vi "Acquisition Message Loop.vi"(8 "error in (no error)":errorcluster, 9 "queue out":refnum<queue>, 10 "Data Notifier":refnum<notifier>, 11 "Message Queues":T1) -> (0 "error out":errorcluster)   [LabVIEW 2018, in "Acquisition.lvlib"]
doc: "Message loop for handling messages pertaining to the acquisition of data from the hardware."
uses:
  Acquisition.lvlib
  support/Message Queue/Message Cluster.ctl
  Acquisition State.ctl
  GlobalVariable/GlobalDisconnected.vi
  GlobalVariable/GlobalFirstRep.vi
  GlobalVariable/GlobalPowerByTime.vi
  GlobalVariable/GlobalPosXbyTime.vi
  GlobalVariable/GlobalPosYbyTime.vi
  GlobalVariable/GlobalProfileByTime.vi
  GlobalVariable/GlobalTensionByTime.vi
  GlobalVariable/GlobalTemperatureByTime.vi
  GlobalVariable/GlobalPredictedPower.vi
  GlobalVariable/Globalt0.vi
  support/Message Queue/Enqueue Message (Single).vi
  GlobalVariable/GlobalLongueurOnde.vi
  GlobalVariable/GlobalTimeStep.vi
  <vilib>/Utility/error.llb/Error Cluster From Error Code.vi
  <vilib>/ErrorRing/Error Ring.xnode
  support/Message Queue/Message Queue.lvlib
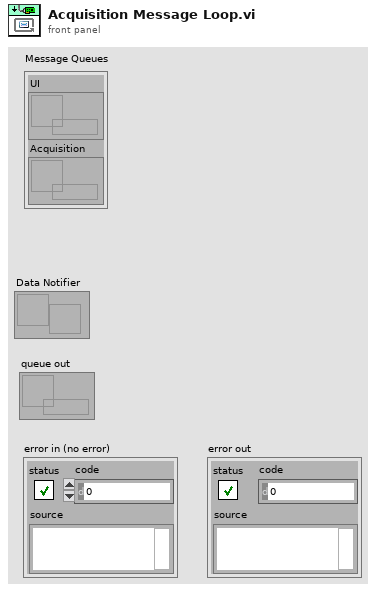
[diagram p1: front panel]
types:
  T1 = cluster{"UI":refnum<queue>, "Acquisition":refnum<queue>}
  T2 = typedef "Acquisition.lvlib/Acquisition State.ctl" = enum16{"Idle", "Acquiring"}
  T3 = enum16{"open", "replace", "create", "open or create", "replace or create", "replace or create with confirmation"}
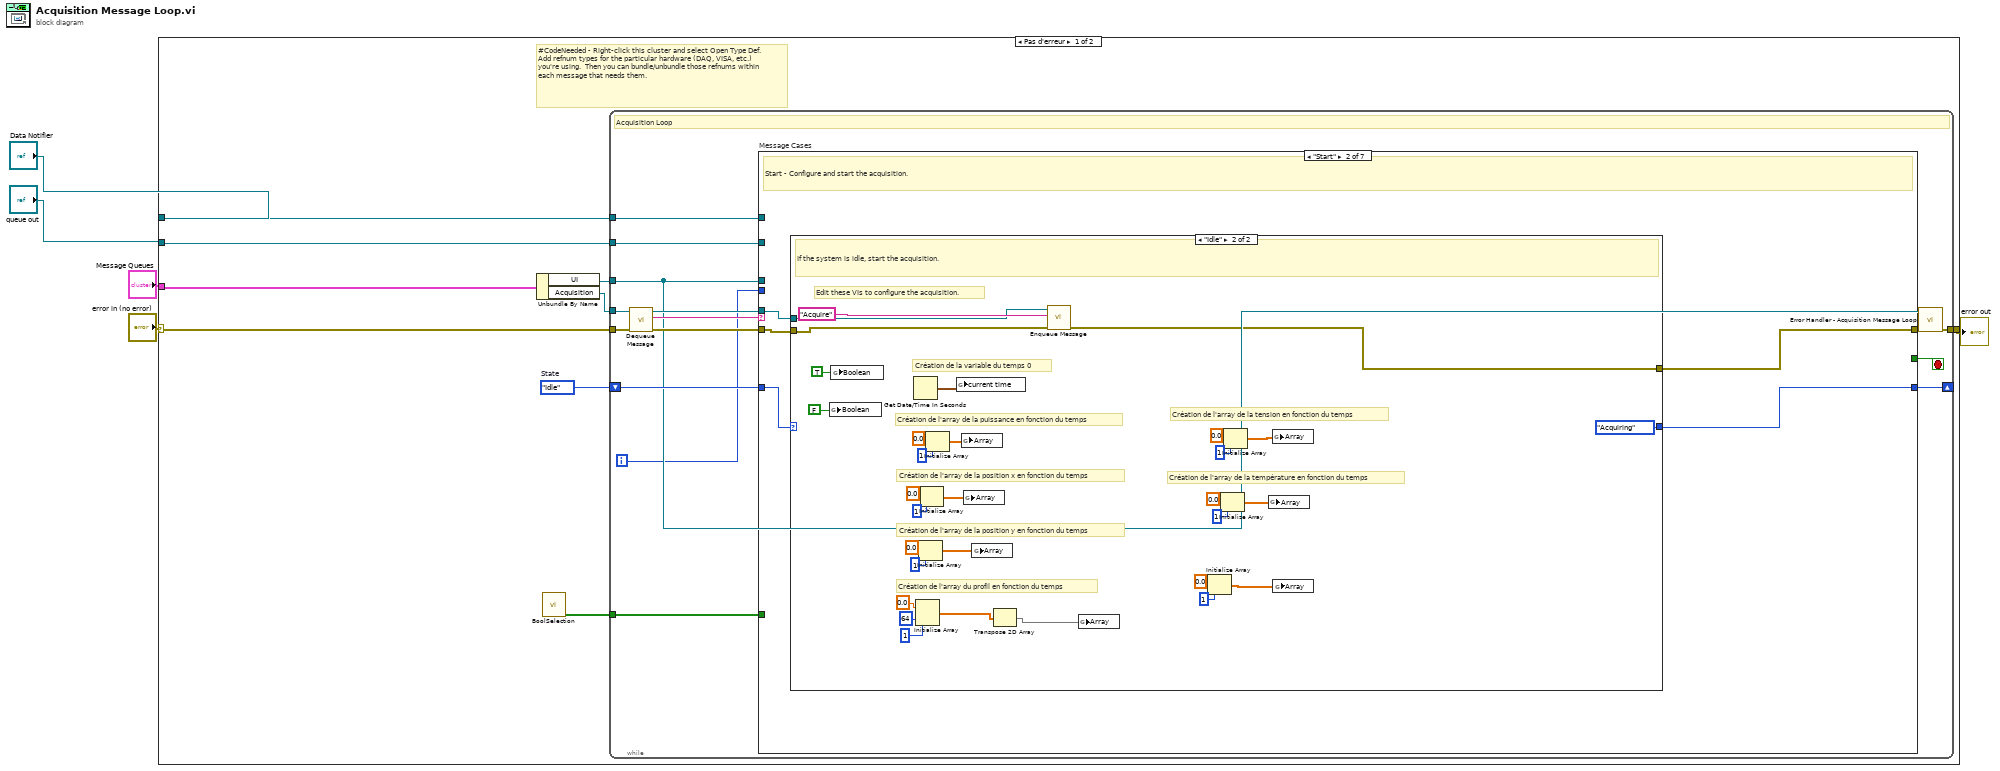
[diagram p0: block diagram]
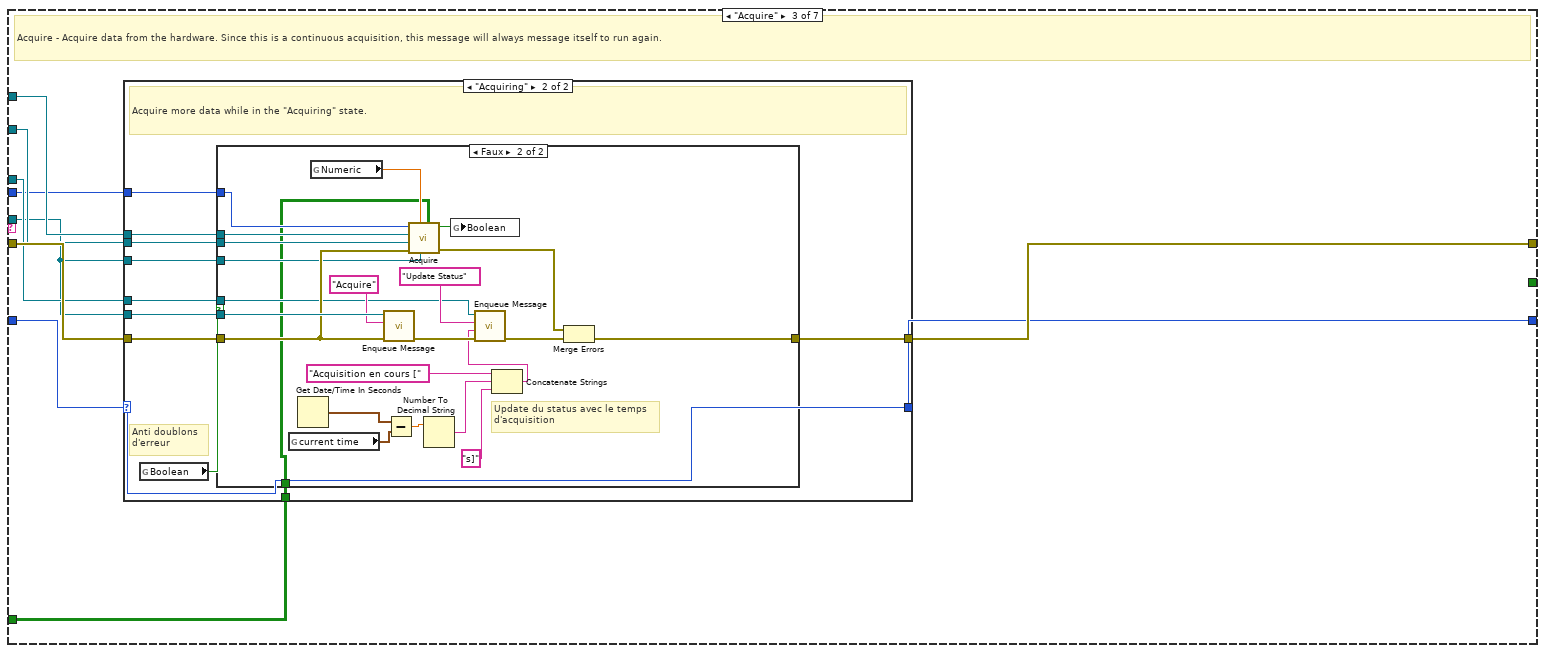
[diagram p4: hidden frame]
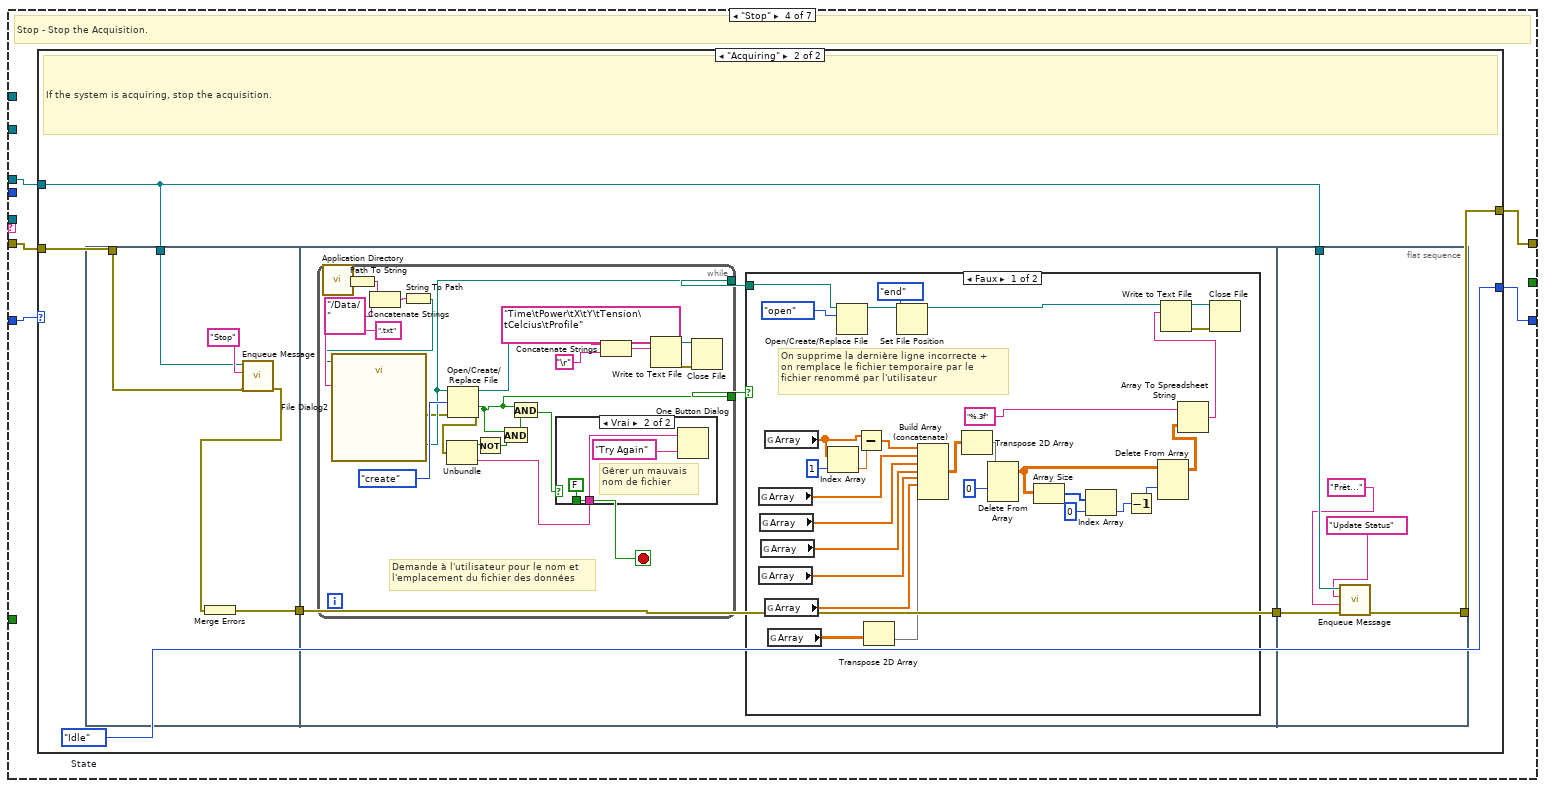
[diagram p7: hidden frame]
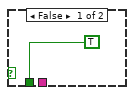
[diagram p10: hidden frame]
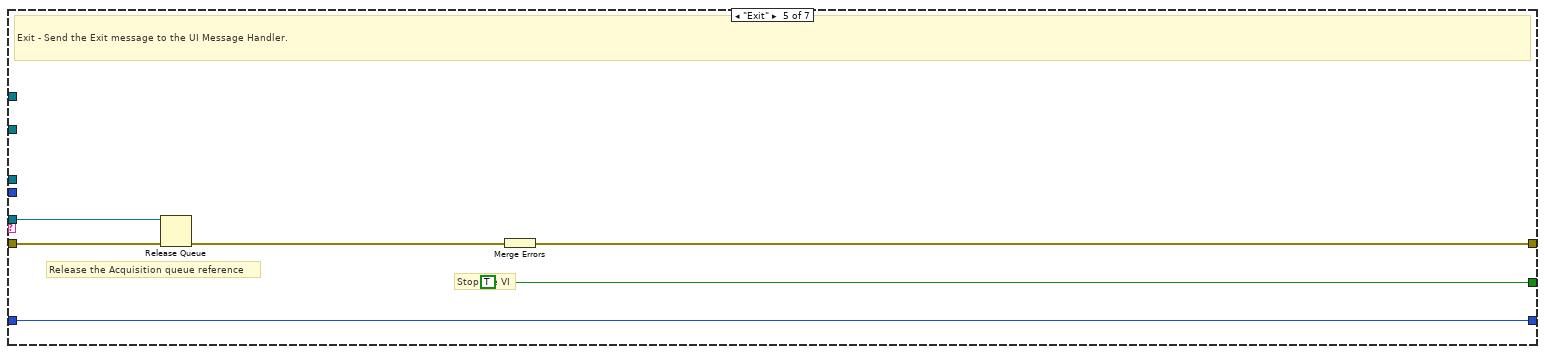
[diagram p11: hidden frame]
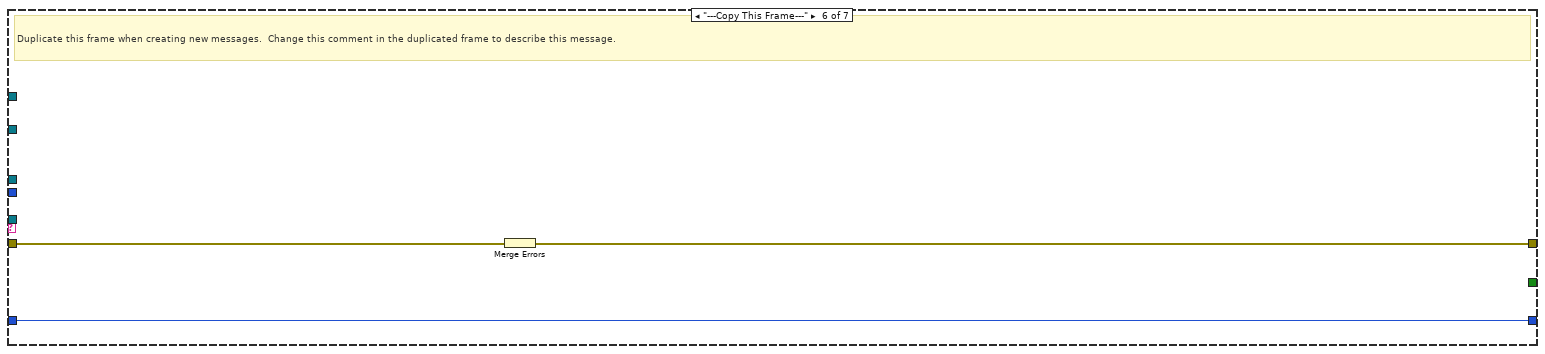
[diagram p12: hidden frame]
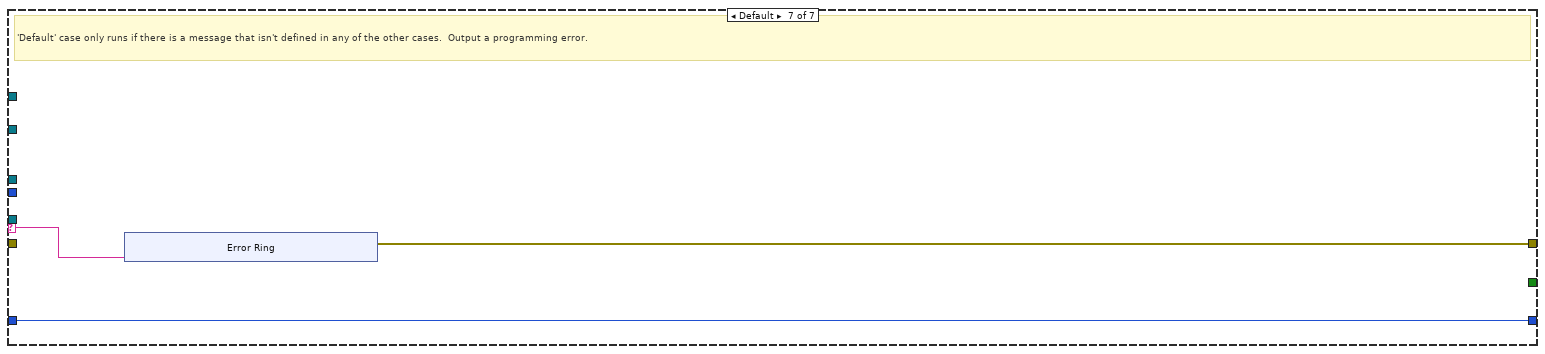
[diagram p13: hidden frame]
diagram:
  n1 = case shown="Pas d'erreur" "error in (no error)" {
    selector: "error in (no error)" -> [w11 w218]
    tunnel: "Message Queues" -> [w14 _]
    tunnel: [w12 w218] -> w4
    tunnel: "Data Notifier" -> [w9 _]
    tunnel: "queue out" -> [w8 _]
    frame No Error {
      w7 = Acquisition_State."Idle"  # State
      # "#CodeNeeded - Right-click this cluster and select Open Type Def.  Add refnum types for the particular hardware (DAQ, VISA, etc.) you're using.  Then you can bundle/unbundle those refnums within each message that needs them."
      n2 = Unbundle By Name(w14) -> ("UI"=w10:refnum<queue>, "Acquisition"=w13:refnum<queue>)
      n3 = call "BoolSelection.vi"() -> ("BoolSelection"=w6:bool[][])  [unwired: 11 in]
      n4 = while {
        tunnel: w13 -> [w17]
        tunnel: w10 -> [w18]
        tunnel: w9 -> [w25]
        tunnel: w8 -> [w24]
        shift-right: [w22] -> _
        shift-left: w7 -> [w23]
        tunnel: w11 -> [w28]
        tunnel: [w21] -> w12
        tunnel: w6 -> [w15]
        i -> [w16]
        stop <- w29 stop-if-true
        # "Acquisition Loop"
        n5 = call "Dequeue Message.vi"("error in (no error)"=w28, "Message Queue"=w17) -> ("error out"=w27:errorcluster, "Message"=w26:string, "dup Message Queue"=w19:refnum<queue>)  [unwired: 6 in, 1 out]
        n6 = case "Message Cases" shown="\"Start\"" w26 {
          selector: w26 -> [_ _ _ _ _ _ w208]
          tunnel: w19 -> [_ w34 w72 _ w200 _ _]
          tunnel: w27 -> [w31 w35 w78 w120 w202 w207 _]
          tunnel: [w31 w36 w79 w118 w203 w206 w209] -> w20
          tunnel: [_ _ _ _ TRUE _ _] -> w29
          tunnel: w18 -> [_ _ w73 w119 _ _ _]
          tunnel: w25 -> [_ _ w77 _ _ _ _]
          tunnel: w24 -> [_ _ w76 _ _ _ _]
          tunnel: w23 -> [w30 w32 w74 w121 w199 w205 w210]
          tunnel: [w30 w33 w75 w117 w199 w205 w210] -> w22
          tunnel: w16 -> [_ _ w71 _ _ _ _]
          tunnel: w15 -> [_ _ w70 _ _ _ _]
          frame "Initialize" {
            # "Initialize  - Initialize is currently a no-op.  The hardware initialization takes place in the 'Start' message."
          }
          frame "Start" {
            # "Start - Configure and start the acquisition."
            n7 = case shown="\"Idle\"" w32 {
              selector: w32 -> [w37 _]
              tunnel: [w38 w65] -> w36
              tunnel: w35 -> [w38 w69]
              tunnel: w34 -> [_ w66]
              tunnel: [w37 Acquisition_State."Acquiring" ("Acquisition State")] -> w33
              frame "Acquiring" {
                # "The system is already acquiring. Ignore the \"Start\" message."
              }
              frame "Idle" {
                # "Création de l'array de la température en fonction du temps"
                # "Création de l'array de la tension en fonction du temps"
                # "Création de la variable du temps 0"
                # "Création de l'array du profil en fonction du temps"
                # "Création de l'array de la position y en fonction du temps"
                # "Création de l'array de la position x en fonction du temps"
                # "Création de l'array de la puissance en fonction du temps"
                # "Edit these VIs to configure the acquisition."
                # "If the system is idle, start the acquisition."
                n8 = global write "GlobalDisconnected.vi" "Boolean"(FALSE) -> ()
                n9 = global write "GlobalFirstRep.vi" "Boolean"(TRUE ("Boolean")) -> ()
                n10 = Get Date/Time In Seconds() -> (seconds since 1Jan1904=w48:timestamp)
                n11 = Initialize Array(0.0, 64 ("dimension size"), 1 ("dimension size")) -> (w61:dbl[][])
                n12 = Initialize Array(0.0, 1) -> (w62:dbl[])
                n13 = Initialize Array(0.0, 1) -> (w63:dbl[])
                n14 = Initialize Array(0.0, 1) -> (w64:dbl[])
                n15 = global write "Globalt0.vi" "current time"(w48) -> ()
                n16 = global write "GlobalPowerByTime.vi" "Array"(w64) -> ()
                n17 = global write "GlobalPosXbyTime.vi" "Array"(w63) -> ()
                n18 = global write "GlobalPosYbyTime.vi" "Array"(w62) -> ()
                n19 = Transpose 2D Array(2D array=w61) -> (transposed array=w60:dbl[][])
                n20 = call-poly "Enqueue Message.vi"("error in (no error)"=w69, "Message"="Acquire", "Message Queue"=w66) -> ("error out"=w65:errorcluster)  [unwired: 7 in, 1 out]
                n21 = global write "GlobalProfileByTime.vi" "Array"(w60) -> ()
                n22 = Initialize Array(0.0, 1) -> (w39:dbl[])
                n23 = Initialize Array(0.0, 1) -> (w42:dbl[])
                n24 = Initialize Array(0.0, 1) -> (w43:dbl[])
                n25 = global write "GlobalTemperatureByTime.vi" "Array"(w42) -> ()
                n26 = global write "GlobalTensionByTime.vi" "Array"(w43) -> ()
                n27 = global write "GlobalPredictedPower.vi" "Array"(w39) -> ()
              }
            }
          }
          frame "Acquire" {
            # "Acquire - Acquire data from the hardware. Since this is a continuous acquisition, this message will always message itself to run again."
            n28 = case shown="\"Acquiring\"" w74 {
              selector: w74 -> [w80 w88]
              tunnel: [w81 w92] -> w79
              tunnel: w72 -> [_ w91]
              tunnel: w78 -> [w81 w87]
              tunnel: w77 -> [_ w90]
              tunnel: w76 -> [_ w89]
              tunnel: [w80 w88] -> w75
              tunnel: w73 -> [_ w86]
              tunnel: w72 -> [_ w85]
              tunnel: w71 -> [_ w83]
              tunnel: w70 -> [_ w82]
              frame "Idle" {
                # "Ignore \"Acquire\" messages when the acquisition is idle."
              }
              frame "Acquiring" {
                # "Anti doublons\nd'erreur"
                # "Acquire more data while in the \"Acquiring\" state."
                n29 = global read "GlobalDisconnected.vi" "Boolean"() -> (w84:bool)
                n30 = case shown="Faux" w84 {
                  tunnel: [w93 w116] -> w92
                  tunnel: w91 -> [_ w115]
                  tunnel: w90 -> [_ w112]
                  tunnel: w89 -> [_ w111]
                  tunnel: w87 -> [w93 w110]
                  tunnel: w86 -> [_ w99]
                  tunnel: w85 -> [_ w98]
                  tunnel: w83 -> [_ w95]
                  tunnel: w82 -> [_ w94]
                  frame True {
                  }
                  frame False {
                    # "Update du status avec le temps\nd'acquisition"
                    n31 = global read "Globalt0.vi" "current time"() -> (w105:timestamp)
                    n32 = Get Date/Time In Seconds() -> (seconds since 1Jan1904=w104:timestamp)
                    n33 = global read "GlobalLongueurOnde.vi" "Numeric"() -> (w97:dbl)
                    n34 = call-poly "Enqueue Message.vi"("error in (no error)"=w110, "Message"="Acquire", "Message Queue"=w115) -> ("error out"=w108:errorcluster)  [unwired: 7 in, 1 out]
                    n35 = Subtract(x=w104, y=w105) -> (x-y=w106:dbl)
                    n36 = call "Acquire.vi"("Bits"=w94, "Acquisition"=w98, "Longueur d'onde"=w97, "error in (no error)"=w110, "Data Queue"=w111, "Data Notifier"=w112, "Loop Count"=w95) -> ("error out"=w114:errorcluster, "Disconnected"=w96:bool)  [unwired: 3 in]
                    n37 = Number To Decimal String(number=w106) -> (decimal integer string=w103:string)  [unwired: 1 in]
                    n38 = global write "GlobalDisconnected.vi" "Boolean"(w96) -> ()
                    n39 = Concatenate Strings("Acquisition en cours [", w103, "s]" ("string")) -> (w101:string)
                    n40 = call-poly "Enqueue Message.vi"("error in (no error)"=w108, "Message Data"=w101, "Message"="Update Status", "Message Queue"=w99) -> ("error out"=w109:errorcluster)  [unwired: 6 in, 1 out]
                    n41 = Merge Errors(w114, w109) -> (w116:errorcluster)
                  }
                }
              }
            }
          }
          frame "Stop" {
            # "Stop - Stop the Acquisition."
            n42 = case shown="\"Acquiring\"" w121 {
              selector: w121 -> [w123 _]
              tunnel: w120 -> [w122 w128]
              tunnel: w119 -> [_ w124]
              tunnel: [w122 w127] -> w118
              tunnel: [w123 w126] -> w117
              frame "Idle" {
                # "The system is already idle. Ignore the \"Stop\" message."
              }
              frame "Acquiring" {
                w126 = Acquisition_State."Idle"  # State
                # "If the system is acquiring, stop the acquisition."
                n43 = flat-sequence {
                  tunnel: [w134] -> w129
                  tunnel: w124 -> [w131]
                  tunnel: w128 -> [w130]
                  tunnel: w129 -> [w136]
                  tunnel: [w136] -> w125
                  tunnel: [w197] -> w127
                  tunnel: w125 -> [w198]
                  tunnel: w124 -> [w196]
                  frame #0 {
                    n44 = call-poly "Enqueue Message.vi"("error in (no error)"=w130, "Message"="Stop", "Message Queue"=w131) -> ("error out"=w133:errorcluster)  [unwired: 7 in, 1 out]
                    n45 = Merge Errors(w133) -> (w134:errorcluster)
                  }
                  frame #1 {
                    n46 = while {
                      tunnel: [w184] -> w137
                      tunnel: [w174] -> w135
                      stop <- w180 stop-if-true
                      # "Demande à l'utilisateur pour le nom et\nl'emplacement du fichier des données"
                      n47 = call <vilib>:"Application Directory.vi"() -> ("Application Directory"=w187:path)
                      n48 = Path To String(path=w187) -> (string=w188:string)
                      n49 = Concatenate Strings(w188, "/Data/") -> (w189:string)
                      n50 = String To Path(string=w189) -> (path=w173:path)
                      n51 = call "File Dialog2"("start path"=w173, "pattern (all files)"=".txt") -> ("selected path"=w184:path, "error out"=w182:errorcluster)  [unwired: 10 in, 2 out]
                      n52 = Open/Create/Replace File(file path (use dialog)=w184, error in=w182, operation (0:open)=T3."create") -> (refnum out=w169:refnum<file>, cancelled=w174:bool, error out=w179:errorcluster)  [unwired: 3 in]
                      n53 = Unbundle(w179) -> ("status"=w178:bool, "source"=w181:string)  [unwired: 1 out]
                      n54 = Not(x=w178) -> (.not. x?=w177:bool)
                      n55 = And(x=w174, y=w177) -> (x .and. y?=w176:bool)
                      n56 = And(x=w174, y=w176) -> (x .and. y?=w175:bool)
                      n57 = case shown="Vrai" w175 {
                        tunnel: w181 -> [_ w193]
                        tunnel: [TRUE FALSE] -> w180
                        frame False {
                        }
                        frame True {
                          # "Gérer un mauvais \nnom de fichier"
                          n58 = One Button Dialog(message=w193, button name ("OK")="Try Again") -> ()  [unwired: 1 out]
                        }
                      }
                      n59 = Concatenate Strings("Time\tPower\tX\tY\tTension\tCelcius\tProfile", "\r") -> (w172:string)
                      n60 = Write to Text File(file (use dialog)=w169, text=w172) -> (refnum out=w168:refnum<file>, error out=w167:errorcluster)  [unwired: 2 in, 1 out]
                      n61 = Close File(refnum=w168, error in=w167) -> ()  [unwired: 2 out]
                    }
                    n62 = case shown="Faux" w135 {
                      tunnel: w137 -> [w160 _]
                      frame False {
                        # "On supprime la dernière ligne incorrecte + \non remplace le fichier temporaire par le \nfichier renommé par l'utilisateur"
                        n63 = global read "GlobalPowerByTime.vi" "Array"() -> (w159:dbl[])
                        n64 = global read "GlobalTensionByTime.vi" "Array"() -> (w139:dbl[])
                        n65 = global read "GlobalPosXbyTime.vi" "Array"() -> (w158:dbl[])
                        n66 = global read "GlobalPosYbyTime.vi" "Array"() -> (w157:dbl[])
                        n67 = global read "GlobalTimeStep.vi" "Array"() -> (w147:dbl[])
                        n68 = global read "GlobalTemperatureByTime.vi" "Array"() -> (w138:dbl[])
                        n69 = global read "GlobalProfileByTime.vi" "Array"() -> (w155:dbl[][])
                        n70 = Index Array(array=w147, index=1) -> (element=w148:dbl)
                        n71 = Open/Create/Replace File(file path (use dialog)=w160, operation (0:open)=T3."open") -> (refnum out=w164:refnum<file>)  [unwired: 4 in, 2 out]
                        n72 = Subtract(x=w147, y=w148) -> (x-y=w146:dbl[])
                        n73 = Transpose 2D Array(2D array=w155) -> (transposed array=w154:dbl[][])
                        n74 = Set File Position(refnum=w164, from (0:start)=enum16{"start", "end", "current"}."end") -> (refnum out=w166:refnum<file>)  [unwired: 2 in, 1 out]
                        n75 = Build Array (concatenate)(w146, w159, w158, w157, w139, w138, w154) -> (w156:dbl[][])
                        n76 = Transpose 2D Array(2D array=w156) -> (transposed array=w150:dbl[][])
                        n77 = Delete From Array(array=w150, index (row)=0) -> (array with subset deleted=w141:dbl[][])  [unwired: 2 in, 1 out]
                        n78 = Array Size(array=w141) -> (size(s)=w145:i32[])
                        n79 = Index Array(array=w145, index=0) -> (element=w143:i32)
                        n80 = Decrement(x=w143) -> (x-1=w142:i32)
                        n81 = Delete From Array(array=w141, index (row)=w142) -> (array with subset deleted=w140:dbl[][])  [unwired: 2 in, 1 out]
                        n82 = Array To Spreadsheet String(array=w140, 3:"%.3f" ("format string")) -> (spreadsheet string=w165:string)  [unwired: 1 in]
                        n83 = Write to Text File(file (use dialog)=w166, text=w165) -> (refnum out=w153:refnum<file>, error out=w152:errorcluster)  [unwired: 2 in, 1 out]
                        n84 = Close File(refnum=w153, error in=w152) -> ()  [unwired: 2 out]
                      }
                      frame True {
                      }
                    }
                  }
                  frame #2 {
                    n85 = call-poly "Enqueue Message.vi"("error in (no error)"=w198, "Message Data"="Prêt...", "Message"="Update Status", "Message Queue"=w196) -> ("error out"=w197:errorcluster)  [unwired: 6 in, 1 out]
                  }
                }
              }
            }
          }
          frame "Exit" {
            # "Release the Acquisition queue reference"
            # "Stop the VI"
            # "Exit - Send the Exit message to the UI Message Handler."
            n86 = Release Queue(queue=w200, error in (no error)=w202) -> (error out=w201:errorcluster)  [unwired: 1 in, 2 out]
            n87 = Merge Errors(w201) -> (w203:errorcluster)
          }
          frame "---Copy This Frame---" {
            # "Duplicate this frame when creating new messages.  Change this comment in the duplicated frame to describe this message."
            n88 = Merge Errors(w207) -> (w206:errorcluster)
          }
          frame Default {
            # "'Default' case only runs if there is a message that isn't defined in any of the other cases.  Output a programming error."
            n89 = xnode "Error Ring"("paramètre 0"=w208) -> ("sortie d'erreur"=w209:errorcluster)
          }
        }
        n90 = call "Error Handler - Acquisition Message Loop.vi"("error in (no error)"=w20, "Message Queue"=w18) -> ("dup error in"=w21:errorcluster)  [unwired: 8 in, 1 out]
      }
    }
    frame Error {
    }
  }
  "error out" <- w4
